vi "MasterAquisitionFile_IOS_US.vi"() -> ()   [LabVIEW 2018]
uses:
  <vilib>/userdefined/High Color/IMAQdx.ctl
  <vilib>/vision/driver/IMAQdx.llb/IMAQdx Camera Control Mode.ctl
  <vilib>/vision/driver/IMAQdx.llb/IMAQdx Acquisition Mode.ctl
  <vilib>/vision/driver/IMAQdx.llb/IMAQdx Buffer Number Mode.ctl
  <vilib>/DAQmx/write.llb/DAQmx Write (Digital Bool 1Line 1Point).vi
  <vilib>/DAQmx/read.llb/DAQmx Read (Analog 1D Wfm NChan NSamp).vi
  <vilib>/DAQmx/write.llb/DAQmx Write (Digital 1D Bool NChan 1Samp 1Line).vi
  <vilib>/DAQmx/create/channels.llb/DAQmx Create Channel (DO-Digital Output).vi
  <vilib>/DAQmx/create/channels.llb/DAQmx Create Channel (CO-Pulse Generation-Frequency).vi
  <vilib>/DAQmx/configure/timing.llb/DAQmx Timing (Implicit).vi
  <vilib>/DAQmx/create/channels.llb/DAQmx Create Channel (AI-Voltage-Basic).vi
  <vilib>/DAQmx/configure/timing.llb/DAQmx Timing (Sample Clock).vi
  <vilib>/DAQmx/configure/trigger.llb/DAQmx Start Trigger (Digital Edge).vi
  <vilib>/DAQmx/miscellaneous.llb/DAQmx Fill In Error Info.vi
  <vilib>/vision/driver/NI_Vision_Acquisition_Software.lvlib
  <resource>/objmgr/imaqdx.rc
panel:
  out "?":T1(plugin-control)
  out "?":T1(plugin-control)
  out "?":T1(plugin-control)
  in  "stop":bool
  out "CBV Cam":bool=TRUE
  out "Whisk Cam":bool=TRUE
  out "Web Cam":bool=TRUE
  out "Analog Data":bool=TRUE
  in  "Physical channels":tag="Dev1/ai0:7"
  out "Web Cam Fs":dbl(knob)=29.663547680668923 scale=0.0..200.0
  out "CBV Cam":dbl(knob)=30.019685039370078 scale=0.0..200.0
  out "Whisk Cam Fs":dbl(knob)=150.04985044865404 scale=0.0..200.0
  in  "Exposure Time (microsec)":string="10000"
  out "Solenoids":bool[](array[boolean])
  out "Analog Samples":i32=18000000
  in  "Analog Channels":string[](array[string])=["Cortical_LH", "Force_Sensor", "LPadSol", "RPadSol", "AudSol", "Hippocampus", "EMG", "Cortical_RH"]
  in  "Whisker Cam ID":T2="cam1"
  in  "WebCam ID":T2="cam0"
  in  "Analog Acquisition":cluster{"Analog Fs":u16}={"Analog Fs"=20000} {"Analog Fs" format="%0.0f"}
  in  "Camera Acquisition Setup":T3={"CBV Cam Fs"=30, "Whisk Cam Fs"=150, "Web Cam Fs"=15, "Pupil Cam Fs"=30}
  out "Notes Size":i32=7
  out "Notes Reversed":string[](array[string])=["Experimenter", "Animal ID", "Hemisphere", "Solenoid PSI", "Isoflurane time", "Session ID", "Amplifier Gain"]
  out "Notes Array":string[](array[string])=["Amplifier Gain", "Session ID", "Isoflurane time", "Solenoid PSI", "Hemisphere", "Animal ID", "Experimenter"]
  in  "Notes:":T4={"Experimenter"="Kevin", "Animal ID"="T119", "Hemisphere"="Both", "Solenoid PSI"="10", "Isoflurane time"="1000", "Session ID"="Imaging Session Six", "Amplifier Gain"="10000"}
  in  "Whisk Cam Trig Source":tag="Dev1/ctr1"
  in  "CBV Cam Trig Source":tag="Dev1/ctr0"
  in  "Right Pad":tag="Dev1/port0/line0"
  in  "Left Pad":tag="Dev1/port0/line1"
  in  "Ultrasound":tag="Dev1/port0/line2"
  in  "Offset (s)":dbl=15.0
  in  "Duration (s)":dbl=0.1 step=0.1
  in  "Interval (s)":dbl=30.0
  in  "Right Pad":dbl=1.0
  in  "Left Pad":dbl=1.0
  in  "Auditory":dbl=1.0
  in  "Target Path":path=path "D:/T119/Imaging Session 6 - 1.29.20" caption="Final saved file location"
  out "Dropped":u32(slide)=135 caption="Whisk Cam" scale=0.0..450.0
  out "Current file name":string="200128_14_10_25"
  out "CBV Camera":bool=TRUE
  out "Time Elapsed (Min)":cluster{dbl, dbl}(slide)={15.0, 15.00305001} scale=0.0..15.0 scale format="%#_2g"
  in  "Time (min)":dbl(knob)=15.0 min=0.5 max=20.0 step=0.5 scale=0.0..20.0 scale format="%#_2g"
  in  "Temp Path":path=path "D:/LabVIEW Streamed Data" caption="Temporary path for streamed data"
  out "Last CBV\nBuffer":i32=27000
  out "Last Whisk\nBuffer":u32=134865
  # "Stimuli"
  # "LPAD"
  # "RPAD"
  # "US"
  # "Whisk Cam ID"
  # "Ratio"
  # "Web Cam ID"
  # "Data Sampling Rates"
  # "Ratio"
  # "Ratio"
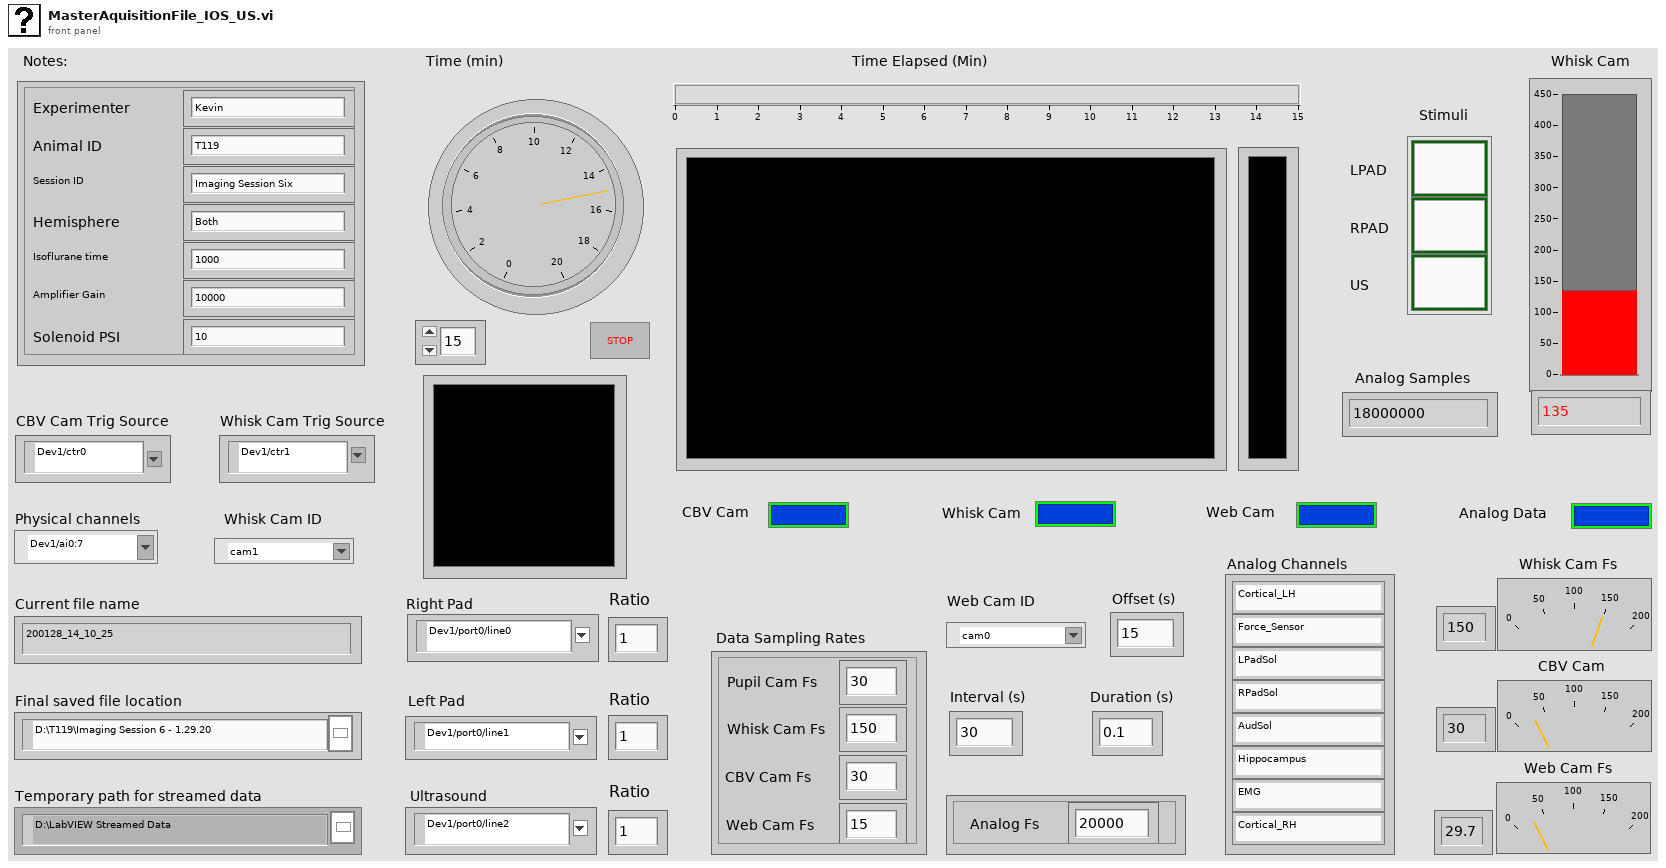
[diagram p1: front panel]
types:
  T1 = typedef "IMAQ Image.ctl" = refnum<image>
  T2 = typedef "IMAQdx.ctl" = refnum<k21>
  T3 = cluster{"CBV Cam Fs":u16, "Whisk Cam Fs":u16, "Web Cam Fs":u16, "Pupil Cam Fs":u16}
  T4 = cluster{"Experimenter":string, "Animal ID":string, "Hemisphere":string, "Solenoid PSI":string, "Isoflurane time":string, "Session ID":string, "Amplifier Gain":string}
  T5 = enum16{"open", "open or create", "create or replace", "create", "open (read-only)"}
  T6 = typedef "Image Type" = u32
  T7 = typedef "NI_Vision_Acquisition_Software.lvlib/IMAQdx Camera Control Mode.ctl" = enum32{"Controller", "Listener"}
  T8 = enum16{"open", "replace", "create", "open or create", "replace or create", "replace or create with confirmation"}
  T9 = typedef "NI_Vision_Acquisition_Software.lvlib/IMAQdx Acquisition Mode.ctl" = enum32{"One Shot", "Continuous"}
  T10 = typedef "IMAQ AVI2 Refnum.ctl" = refnum<k20>
  T11 = enum16{"big-endian, network order", "native, host order", "little-endian"}
  T12 = typedef "NI_Vision_Acquisition_Software.lvlib/IMAQdx Buffer Number Mode.ctl" = enum32{"Next", "Last", "Buffer Number", "Every", "Last New"}
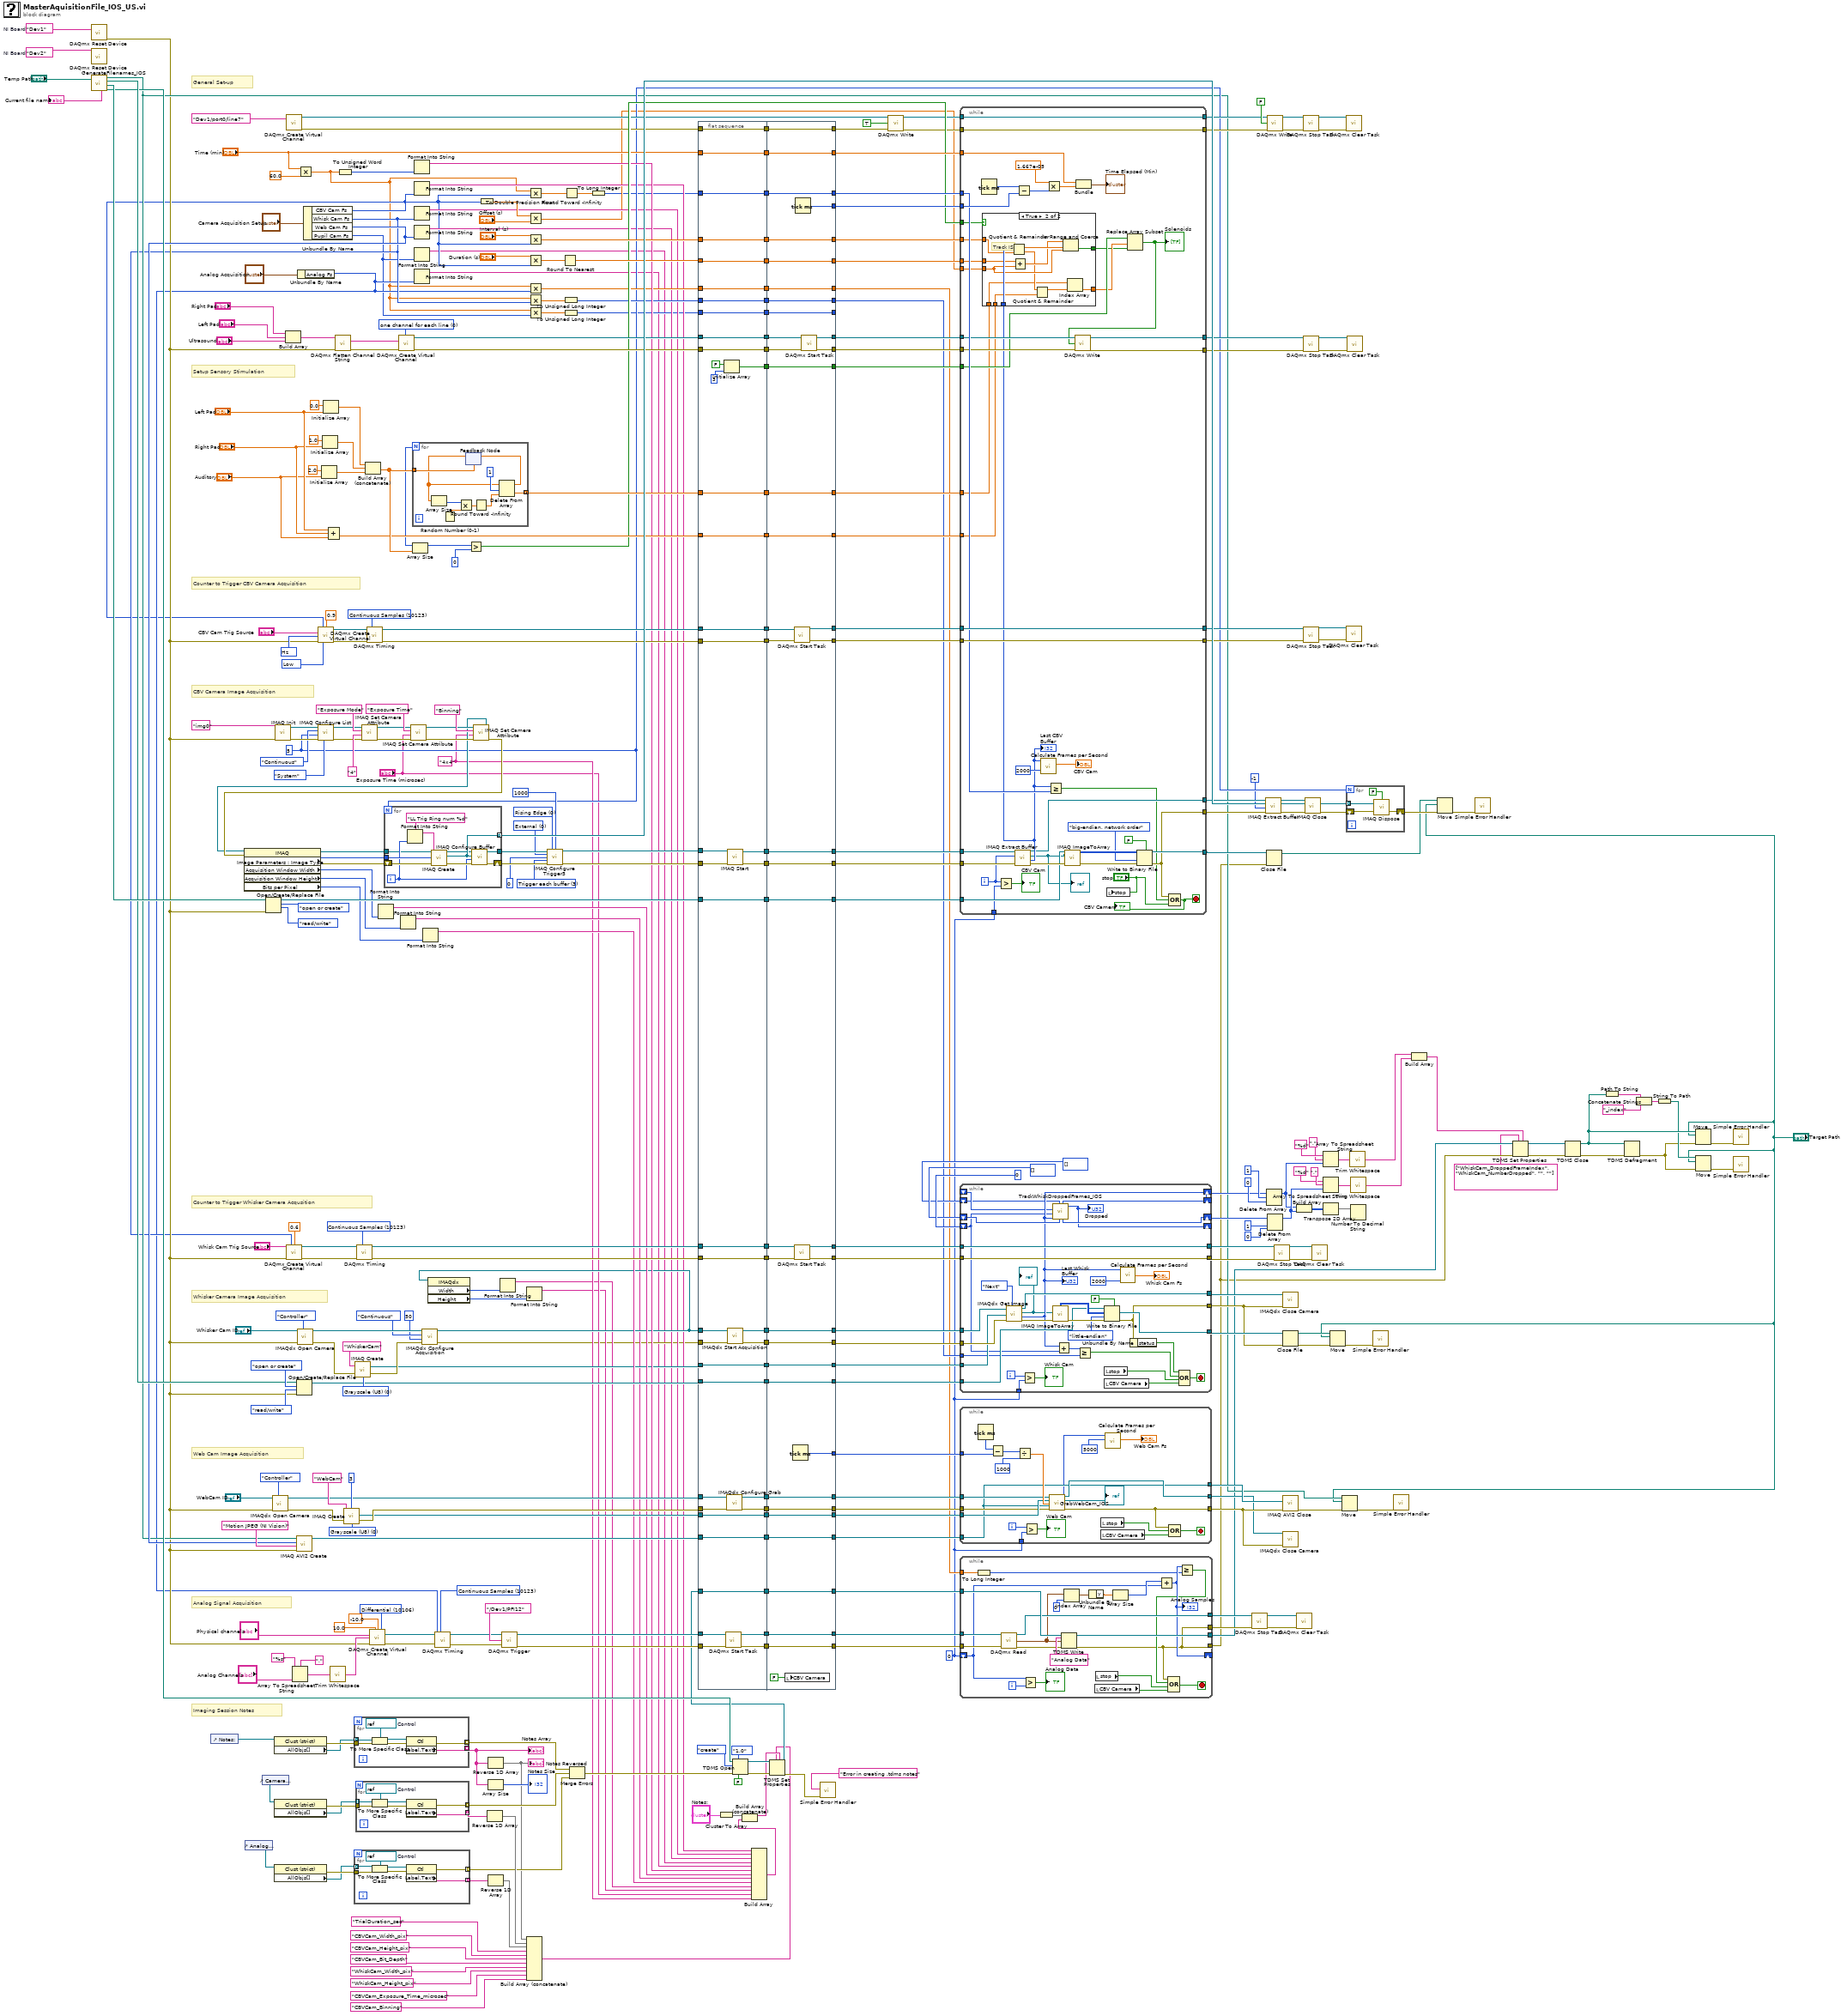
[diagram p0: block diagram]
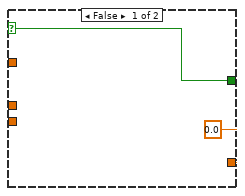
[diagram p2: hidden frame]
diagram:
  w16 = tag "Dev2"  # NI Board
  w48 = "4x4" ("Attribute Value")
  w22 = 0
  w207 = 0 items=["one channel for each line", "one channel for all lines"] ("line grouping")
  w260 = 10123 items=["Finite Samples"=10178, "Continuous Samples"=10123, "Hardware Timed Single Point"=12522] ("sample mode")
  w263 = 10106 items=["default"=-1, "RSE"=10083, "NRSE"=10078, "Differential"=10106, "Pseudodifferential"=12529] ("input terminal configuration")
  w314 = T6 0 items=["Grayscale (U8)", "Grayscale (I16)", "Grayscale (SGL)", "Complex (CSG)", "RGB (U32)", "HSL (U32)", "RGB (U64)", "Grayscale (U16)"] ("Image Type")
  w334 = u32 0 items=["Rising Edge", "Falling Edge"] ("Trigger Polarity")
  w337 = u32 0 items=["External"=0, "RTSI"=1, "ISO In"=2, "Scaled Encoder"=5] ("Trigger Type")
  w328 = tag "Dev1"  # NI Board
  w329 = 10123 items=["Finite Samples"=10178, "Continuous Samples"=10123, "Hardware Timed Single Point"=12522] ("sample mode")
  w332 = 10373 items=["Hz"=10373] ("units")
  w333 = 10214 items=["High"=10192, "Low"=10214] ("idle state")
  w53 = u32 5 ("Number of Buffers")
  w335 = u32 3 items=["Disabled", "Trigger start of acquisition", "Trigger start of each buffer list", "Trigger each buffer", "Trigger each line (linescan)", "Trigger end of acquisition"] ("Action")
  w349 = 10123 items=["Finite Samples"=10178, "Continuous Samples"=10123, "Hardware Timed Single Point"=12522] ("sample mode")
  w356 = T6 0 items=["Grayscale (U8)", "Grayscale (I16)", "Grayscale (SGL)", "Complex (CSG)", "RGB (U32)", "HSL (U32)", "RGB (U64)", "Grayscale (U16)"] ("Image Type")
  # "General Set-up"
  # "Whisker Camera Image Acquisition"
  # "Imaging Session Notes"
  # "Setup Sensory Stimulation"
  # "CBV Camera Image Acquisition"
  # "Counter to Trigger CBV Camera Acquisition"
  # "Counter to Trigger Whisker Camera Acqusition"
  # "Web Cam Image Acquisition"
  # "Analog Signal Acquisition"
  n1 = call <vilib>:"DAQmx Reset Device.vi"("device in"=w328) -> ("error out"=w44:errorcluster)  [unwired: 14 in]
  n2 = call <vilib>:"DAQmx Reset Device.vi"("device in"=w16) -> ()  [unwired: 14 in, 1 out]
  n3 = call "GenerateFilenames_IOS.vi"("path"="Temp Path") -> ("TDMS Path"=w163:path, "Dalsa Path"=w321:path, "Basler Path"=w317:path, "WebCam Path"=w52:path, "Analog file name"=→"Current file name":string)  [unwired: 3 in, 3 out]
  n4 = control-ref of="Notes:"() -> (w168:refnum<vi>)
  n5 = control-ref of="Analog Acquisition"() -> (w146:refnum<vi>)
  n6 = control-ref of="Camera Acquisition Setup"() -> (w147:refnum<vi>)
  n7 = Open/Create/Replace File(file path (use dialog)=w321, error in=w44, operation (0:open)=T8."open or create", access (0:read/write)=enum16{"read/write", "read-only", "write-only"}."read/write") -> (refnum out=w264:refnum<file>)  [unwired: 2 in, 2 out]
  n8 = call <vilib>:"IMAQdx Open Camera.vi"("Camera Control Mode"=IMAQdx_Camera_Control_Mode."Controller", "error in"=w44, "Session In"="WebCam ID") -> ("error out"=w310:errorcluster, "Session Out"=w308:T2)  [unwired: 7 in]
  n9 = property class="Clust (strict)"(reference=w168) -> (error out=w171:errorcluster, "AllObjs[]"=w60:refnum<vi>[])  [unwired: 1 in, 1 out]
  n10 = property class="Clust (strict)"(reference=w147) -> (error out=w166:errorcluster, "AllObjs[]"=w61:refnum<vi>[])  [unwired: 1 in, 1 out]
  n11 = property class="Clust (strict)"(reference=w146) -> (error out=w145:errorcluster, "AllObjs[]"=w59:refnum<vi>[])  [unwired: 1 in, 1 out]
  n12 = call <vilib>:"IMAQ Init.vi"("error in (no error)"=w44, "Interface Name"="img0") -> ("error out"=w347:errorcluster, "IMAQ Session Out"=w348:refnum<k11>)  [unwired: 8 out]
  n13 = Build Array("Right Pad", "Left Pad", "Ultrasound") -> (w11:tag[])
  n14 = call-poly <vilib>:"DAQmx Create Virtual Channel.vi"("lines"=tag "Dev1/port0/line7") -> ("task out"=w93:refnum<k21>, "error out"=w96:errorcluster)  [unwired: 13 in]
  n15 = Array To Spreadsheet String(delimiter (Tab)=",", array="Analog Channels", 3:"%s" ("format string")) -> (spreadsheet string=w132:string)
  n16 = Open/Create/Replace File(file path (use dialog)=w317, error in=w44, operation (0:open)=T8."open or create", access (0:read/write)=enum16{"read/write", "read-only", "write-only"}."read/write") -> (refnum out=w282:refnum<file>)  [unwired: 2 in, 2 out]
  n17 = Unbundle By Name("Analog Acquisition") -> ("Analog Fs"=w37:u16)
  n18 = call <vilib>:"IMAQdx Open Camera.vi"("Camera Control Mode"=IMAQdx_Camera_Control_Mode."Controller", "error in"=w44, "Session In"="Whisker Cam ID") -> ("error out"=w359:errorcluster, "Session Out"=w362:T2)  [unwired: 7 in]
  n19 = Multiply(x="Time (min)", y=60.0) -> (x*y=w24:dbl)
  n20 = Unbundle By Name("Camera Acquisition Setup") -> ("CBV Cam Fs"=w26:u16, "Whisk Cam Fs"=w42:u16, "Web Cam Fs"=w140:u16, "Pupil Cam Fs"=w35:u16)
  n21 = call-poly <vilib>:"DAQmx Create Virtual Channel.vi"("frequency"=w42, "duty cycle"=0.6, "counter"="Whisk Cam Trig Source", "error in"=w44) -> ("task out"=w351:refnum<k21>, "error out"=w350:errorcluster)  [unwired: 10 in]
  n22 = call "IMAQ AVI2 Create"("error in (no error)"=w44, "Codec"="Motion JPEG (NI Vision)", "Frames Per Second"=w140, "AVI Path"=w52) -> ("AVI Refnum"=w300:T10)  [unwired: 6 in, 1 out]
  n23 = call <vilib>:"IMAQ Configure List.vi"("Memory Location"=enum16{"System", "Onboard"}."System", "error in (no error)"=w347, "Number of buffers"=w53, "Continuous?"=enum16{"One-Shot", "Continuous"}."Continuous" ("Continuous ?"), "IMAQ Session In"=w348) -> ("error out"=w74:errorcluster, "IMAQ Session Out"=w70:refnum<k11>)  [unwired: 1 in, 4 out]
  n24 = call-poly <vilib>:"DAQmx Create Virtual Channel.vi"("frequency"=w26, "duty cycle"=0.9, "counter"="CBV Cam Trig Source", "units"=w332, "error in"=w44, "idle state"=w333) -> ("task out"=w331:refnum<k21>, "error out"=w330:errorcluster)  [unwired: 8 in]
  n25 = Initialize Array(2.0 ("element"), "Auditory") -> (w20:dbl[])
  n26 = Initialize Array(1.0 ("element"), "Right Pad") -> (w211:dbl[])
  n27 = Initialize Array(0.0 ("element"), "Left Pad") -> (w212:dbl[])
  n28 = Compound Arithmetic op=ADD("Left Pad", "Right Pad", "Auditory") -> (w191:dbl)
  n29 = call <vilib>:"Trim Whitespace.vi"("string"=w132) -> ("trimmed string"=w131:string)  [unwired: 1 in]
  n30 = call <vilib>:"DAQmx Flatten Channel String.vi"("names in"=w11, "error in"=w44) -> ("names out"=w173:string, "error out"=w172:errorcluster)  [unwired: 12 in]
  n31 = To Unsigned Word Integer(number=w24) -> (unsigned 16bit integer=w126:u16)
  n32 = call "IMAQ Create"("Border Size"=3, "Image Name"="WebCam", "Image Type"=w314, "error in (no error)"=w310) -> ("New Image"=w307:T1, "error out"=w309:errorcluster)  [unwired: 1 in]
  n33 = for {
    tunnel: [w368] -> w170 mode=indexing
    tunnel: w171 -> [w367]
    tunnel: [w365] -> w154 mode=indexing
    tunnel: w60 -> [w364] mode=indexing
    w369 = refnum<vi> refnum  # Control
    n34 = To More Specific Class(target class=w369, reference=w364, error in=w367) -> (specific class reference=w370:refnum<vi>, error out=w366:errorcluster)
    n35 = property class="Ctl"(reference=w370, error in=w366) -> (error out=w365:errorcluster, "Label.Text"=w368:string)  [unwired: 1 out]
  }
  "Notes Array" <- w170
  n36 = for {
    tunnel: [w375] -> w143 mode=indexing
    tunnel: w145 -> [w374]
    tunnel: [w372] -> w144 mode=indexing
    tunnel: w59 -> [w371] mode=indexing
    w376 = refnum<vi> refnum  # Control
    n37 = To More Specific Class(target class=w376, reference=w371, error in=w374) -> (specific class reference=w377:refnum<vi>, error out=w373:errorcluster)
    n38 = property class="Ctl"(reference=w377, error in=w373) -> (error out=w372:errorcluster, "Label.Text"=w375:string)  [unwired: 1 out]
  }
  n39 = call "IMAQ Create"("Image Name"="WhiskerCam", "Image Type"=w356, "error in (no error)"=w359) -> ("New Image"=w113:T1, "error out"=w357:errorcluster)  [unwired: 2 in]
  n40 = for {
    tunnel: [w382] -> w167 mode=indexing
    tunnel: w166 -> [w381]
    tunnel: [w379] -> w153 mode=indexing
    tunnel: w61 -> [w378] mode=indexing
    w383 = refnum<vi> refnum  # Control
    n41 = To More Specific Class(target class=w383, reference=w378, error in=w381) -> (specific class reference=w384:refnum<vi>, error out=w380:errorcluster)
    n42 = property class="Ctl"(reference=w384, error in=w380) -> (error out=w379:errorcluster, "Label.Text"=w382:string)  [unwired: 1 out]
  }
  n43 = call-poly <vilib>:"DAQmx Timing.vi"("task/channels in"=w351, "sample mode"=w349, "error in"=w350) -> ("task out"=w243:refnum<k21>, "error out"=w241:errorcluster)  [unwired: 11 in]
  n44 = call <vilib>:"IMAQ Set Camera Attribute.vi"("error in (no error)"=w74, "Attribute Value"="4", "Camera Attribute"="Exposure Mode", "IMAQ Session In"=w70) -> ("error out"=w73:errorcluster, "IMAQ Session Out"=w69:refnum<k11>)  [unwired: 4 in]
  n45 = Build Array (concatenate)(w212, w211, w20) -> (w210:dbl[])
  n46 = call-poly <vilib>:"DAQmx Timing.vi"("task/channels in"=w331, "sample mode"=w329, "error in"=w330) -> ("task out"=w247:refnum<k21>, "error out"=w245:errorcluster)  [unwired: 11 in]
  n47 = call-poly <vilib>:"DAQmx Create Virtual Channel.vi"("maximum value"=10.0, "minimum value"=-10.0, "input terminal configuration"=w263, "physical channels"="Physical channels", "name to assign"=w131, "error in"=w44) -> ("task out"=w262:refnum<k21>, "error out"=w261:errorcluster)  [unwired: 8 in]
  n48 = call-poly <vilib>:"DAQmx Create Virtual Channel.vi"("lines"=w173, "line grouping"=w207, "error in"=w172) -> ("task out"=w205:refnum<k21>, "error out"=w203:errorcluster)  [unwired: 11 in]
  n49 = call <vilib>:"IMAQ Set Camera Attribute.vi"("error in (no error)"=w73, "Attribute Value"="Exposure Time (microsec)", "Camera Attribute"="Exposure Time", "IMAQ Session In"=w69) -> ("error out"=w72:errorcluster, "IMAQ Session Out"=w68:refnum<k11>)  [unwired: 4 in]
  n50 = Array Size(array=w210) -> (size(s)=w137:i32)
  n51 = for {
    N: w137 -> [_]
    tunnel: w210 -> [w388]
    tunnel: [w385] -> w188 mode=concatenating
    n52 = Random Number (0-1)() -> (number: 0 to 1=w392:dbl)
    n53 = feedback #1(w388) -> (w387:dbl[])
    n54 = Array Size(array=w387) -> (size(s)=w393:i32)
    n55 = Multiply(x=w393, y=w392) -> (x*y=w391:dbl)
    n56 = Round Toward -Infinity(1:w391) -> (0:w390:dbl)
    n57 = Delete From Array(array=w387, length=1, index=w390) -> (deleted portion=w385:dbl[], array with subset deleted=w386:dbl[])
    n58 = feedback-in #1(w386) -> ()
  }
  n59 = Format Into String(w126) -> (resulting string=w128:string)  [unwired: 3 in, 1 out]
  n60 = Format Into String(w26) -> (resulting string=w40:string)  [unwired: 3 in, 1 out]
  n61 = Format Into String(w42) -> (resulting string=w39:string)  [unwired: 3 in, 1 out]
  n62 = Format Into String(w140) -> (resulting string=w38:string)  [unwired: 3 in, 1 out]
  n63 = Format Into String(w35) -> (resulting string=w6:string)  [unwired: 3 in, 1 out]
  n64 = Format Into String(w37) -> (resulting string=w5:string)  [unwired: 3 in, 1 out]
  n65 = call <vilib>:"IMAQdx Configure Acquisition.vi"("error in"=w357, "Number of Buffers"=u32 50, "Continuous?"=IMAQdx_Acquisition_Mode."Continuous", "Session In"=w362) -> ("error out"=w23:errorcluster, "Session Out"=w114:T2)  [unwired: 6 in]
  n66 = property class="IMAQdx"(reference=w114) -> ("Width"=w125:u32, "Height"=w124:u32)  [unwired: 1 in, 2 out]
  n67 = call-poly <vilib>:"DAQmx Timing.vi"("task/channels in"=w262, "sample mode"=w260, "rate"=w37, "error in"=w261) -> ("task out"=w57:refnum<k21>, "error out"=w259:errorcluster)  [unwired: 10 in]
  n68 = Greater?(x=w137, y=0) -> (0:w135:bool)
  n69 = call <vilib>:"IMAQ Set Camera Attribute.vi"("error in (no error)"=w72, "Attribute Value"=w48, "Camera Attribute"="Binning", "IMAQ Session In"=w68) -> ("error out"=w71:errorcluster, "IMAQ Session Out"=w67:refnum<k11>)  [unwired: 4 in]
  n70 = property class="IMAQ"(reference=w67, error in=w71) -> (reference out=w81:refnum<k11>, error out=w80:errorcluster, "Image Parameters : Image Type"=w343:u32, "Acquisition Window Width"=w123:u32, "Acquisition Window Height"=w122:u32, "Bits per Pixel"=w121:u32)
  n71 = Format Into String(w123) -> (resulting string=w120:string)  [unwired: 3 in, 1 out]
  n72 = for {
    N: w53 -> [_]
    tunnel: [w403] -> w339
    tunnel: w343 -> [w401]
    shift-right: [w402] -> w338
    shift-left: w80 -> [w400]
    tunnel: [w395] -> w340 mode=indexing
    tunnel: w81 -> [w394]
    i -> [w396]
    n73 = Format Into String(format string="LL Trig Ring num %d", w396) -> (resulting string=w398:string)  [unwired: 2 in, 1 out]
    n74 = call "IMAQ Create"("Image Name"=w398, "Image Type"=w401, "error in (no error)"=w400) -> ("New Image"=w395:T1, "error out"=w399:errorcluster)  [unwired: 1 in, 1 out]
    n75 = call <vilib>:"IMAQ Configure Buffer.vi"("error in (no error)"=w399, "Buffer Number"=w396, "Image In"=w395, "IMAQ Session In"=w394) -> ("error out"=w402:errorcluster, "IMAQ Session Out"=w403:refnum<k11>)  [unwired: 2 in, 4 out]
  }
  n76 = Format Into String(w122) -> (resulting string=w54:string)  [unwired: 3 in, 1 out]
  n77 = Format Into String(w121) -> (resulting string=w119:string)  [unwired: 3 in, 1 out]
  n78 = To Double Precision Float(number=w26) -> (double precision float=w174:dbl)
  n79 = Reverse 1D Array(array=w167) -> (reversed array=w157:string[])
  n80 = Reverse 1D Array(array=w170) -> (reversed array=w58:string[])
  "Notes Reversed" <- w58
  n81 = Array Size(array=w170) -> (size(s)=→"Notes Size":i32)
  n82 = Reverse 1D Array(array=w143) -> (reversed array=w142:string[])
  n83 = Format Into String(w125) -> (resulting string=w45:string)  [unwired: 3 in, 1 out]
  n84 = call-poly <vilib>:"DAQmx Trigger.vi"("task/channels in"=w57, "source"=tag "/Dev1/PFI12", "error in"=w259) -> ("task out"=w257:refnum<k21>, "error out"=w256:errorcluster)  [unwired: 11 in]
  n85 = Build Array (concatenate)(w58, w157, w142, "TrialDuration_sec", "CBVCam_Width_pix", "CBVCam_Height_pix", "CBVCam_Bit_Depth", "WhiskCam_Width_pix", "WhiskCam_Height_pix", "CBVCam_Exposure_Time_microsec" ("element"), "CBVCam_Binning" ("element")) -> (w49:string[])
  n86 = Format Into String(w124) -> (resulting string=w46:string)  [unwired: 3 in, 1 out]
  n87 = Multiply(x=w24, y=w26) -> (x*y=w319:dbl)
  n88 = Multiply(x="Offset (s)", y=w174) -> (x*y=w33:dbl)
  n89 = Multiply(x="Interval (s)", y=w26) -> (x*y=w195:dbl)
  n90 = Multiply(x="Duration (s)", y=w26) -> (x*y=w182:dbl)
  n91 = Multiply(x=w24, y=w37) -> (x*y=w102:dbl)
  n92 = Multiply(x=w42, y=w24) -> (x*y=w55:dbl)
  n93 = Multiply(x=w35, y=w24) -> (x*y=w41:dbl)
  n94 = call <vilib>:"IMAQ Configure Trigger3.vi"("IMAQ Session In"=w339, "Polarity"=w334, "Frame timeout (ms)"=u32 1000 ("Frame Timeout (ms)"), "Type"=w337, "Line Number"=u32 0 ("Trigger Line Number"), "Action"=w335, "error in (no error)"=w338) -> ("IMAQ Session Out"=w281:refnum<k11>, "error out"=w280:errorcluster)  [unwired: 2 in, 5 out]
  n95 = Round To Nearest(number=w182) -> (nearest integer value=w181:dbl)
  n96 = To Unsigned Long Integer(number=w55) -> (unsigned 32bit integer=w100:u32)
  n97 = To Unsigned Long Integer(number=w41) -> (unsigned 32bit integer=w36:u32)
  n98 = Round Toward -Infinity(1:w319) -> (0:w318:dbl)
  n99 = Merge Errors(w154, w153, w144) -> (w152:errorcluster)
  n100 = To Long Integer(number=w318) -> (32bit integer=w25:i32)
  n101 = flat-sequence {
    tunnel: w309 -> [w444]
    tunnel: w308 -> [w443]
    tunnel: w307 -> [w442]
    tunnel: [w442] -> w306
    tunnel: [w441] -> w304
    tunnel: [w440] -> w302
    tunnel: w300 -> [w439]
    tunnel: [w439] -> w299
    tunnel: w114 -> [w438]
    tunnel: w23 -> [w437]
    tunnel: [w436] -> w289
    tunnel: [w435] -> w287
    tunnel: [w434] -> w285
    tunnel: w113 -> [w434]
    tunnel: [w433] -> w283
    tunnel: w282 -> [w433]
    tunnel: w281 -> [w432]
    tunnel: w280 -> [w431]
    tunnel: [w430] -> w278
    tunnel: [w429] -> w276
    tunnel: w25 -> [w428]
    tunnel: [w428] -> w270
    tunnel: "Time (min)" -> [w427]
    tunnel: [w427] -> w267
    tunnel: [w426] -> w265
    tunnel: w264 -> [w426]
    tunnel: w257 -> [w425]
    tunnel: w256 -> [w424]
    tunnel: [w423] -> w255
    tunnel: [w422] -> w254
    tunnel: [w421] -> w249
    tunnel: w155 -> [w421]
    tunnel: w247 -> [w420]
    tunnel: [w420] -> w246
    tunnel: w245 -> [w419]
    tunnel: [w419] -> w244
    tunnel: w243 -> [w418]
    tunnel: [w418] -> w242
    tunnel: w241 -> [w417]
    tunnel: [w417] -> w240
    tunnel: w205 -> [w416]
    tunnel: [w416] -> w206
    tunnel: w203 -> [w415]
    tunnel: [w415] -> w204
    tunnel: w195 -> [w414]
    tunnel: [w414] -> w194
    tunnel: [w413] -> w192
    tunnel: w181 -> [w413]
    tunnel: w191 -> [w412]
    tunnel: [w412] -> w190
    tunnel: w188 -> [w411]
    tunnel: [w411] -> w187
    tunnel: [w409] -> w185
    tunnel: w102 -> [w407]
    tunnel: [w407] -> w101
    tunnel: w100 -> [w406]
    tunnel: [w406] -> w99
    tunnel: w96 -> [w405]
    tunnel: [w405] -> w95
    tunnel: w36 -> [w404]
    tunnel: [w404] -> w34
    tunnel: [w484] -> w311
    tunnel: w306 -> [w483]
    tunnel: [w483] -> w305
    tunnel: w304 -> [w482]
    tunnel: [w482] -> w303
    tunnel: w302 -> [w481]
    tunnel: [w481] -> w301
    tunnel: w299 -> [w480]
    tunnel: [w480] -> w298
    tunnel: [w462] -> w295
    tunnel: [w461] -> w293
    tunnel: [w479] -> w290
    tunnel: w289 -> [w479]
    tunnel: [w478] -> w288
    tunnel: w287 -> [w478]
    tunnel: [w477] -> w286
    tunnel: w285 -> [w477]
    tunnel: [w476] -> w284
    tunnel: w283 -> [w476]
    tunnel: [w475] -> w279
    tunnel: w278 -> [w475]
    tunnel: [w474] -> w277
    tunnel: w276 -> [w474]
    tunnel: [w466] -> w274
    tunnel: [w465] -> w272
    tunnel: [w473] -> w271
    tunnel: w270 -> [w472]
    tunnel: [w472] -> w269
    tunnel: [w471] -> w268
    tunnel: w267 -> [w471]
    tunnel: [w470] -> w266
    tunnel: w265 -> [w470]
    tunnel: [w469] -> w252
    tunnel: w255 -> [w469]
    tunnel: [w468] -> w253
    tunnel: w254 -> [w468]
    tunnel: [w467] -> w250
    tunnel: w249 -> [w467]
    tunnel: w246 -> [w464]
    tunnel: w244 -> [w463]
    tunnel: w242 -> [w460]
    tunnel: w240 -> [w459]
    tunnel: w206 -> [w458]
    tunnel: w204 -> [w457]
    tunnel: [w456] -> w202
    tunnel: [w455] -> w201
    tunnel: [w454] -> w196
    tunnel: w194 -> [w454]
    tunnel: [w453] -> w193
    tunnel: w192 -> [w453]
    tunnel: w190 -> [w452]
    tunnel: [w452] -> w189
    tunnel: w187 -> [w451]
    tunnel: [w451] -> w186
    tunnel: w185 -> [w450]
    tunnel: [w450] -> w184
    tunnel: w101 -> [w449]
    tunnel: [w449] -> w31
    tunnel: w99 -> [w448]
    tunnel: [w448] -> w32
    tunnel: w95 -> [w447]
    tunnel: [w447] -> w94
    tunnel: [w445] -> _
    tunnel: w34 -> [w445]
    frame #0 {
      n102 = Initialize Array(FALSE, 3 ("dimension size")) -> (w409:bool[])
      n103 = call <vilib>:"DAQmx Start Task.vi"("task/channels in"=w425, "error in"=w424) -> ("task out"=w423:refnum<k21>, "error out"=w422:errorcluster)  [unwired: 12 in]
      n104 = call <vilib>:"IMAQdx Configure Grab.vi"("error in"=w444, "Session In"=w443) -> ("error out"=w440:errorcluster, "Session Out"=w441:T2)  [unwired: 8 in]
      n105 = call <vilib>:"IMAQ Start.vi"("error in (no error)"=w431, "IMAQ Session In"=w432) -> ("error out"=w429:errorcluster, "IMAQ Session Out"=w430:refnum<k11>)  [unwired: 8 out]
      n106 = call <vilib>:"IMAQdx Start Acquisition.vi"("error in"=w437, "Session In"=w438) -> ("error out"=w435:errorcluster, "Session Out"=w436:T2)  [unwired: 8 in]
    }
    frame #1 {
      n107 = local write "CBV Camera"(FALSE ("Finished Acquiring")) -> ()
      n108 = Tick Count (ms)() -> (millisecond timer value=w484:u32)
      n109 = call <vilib>:"DAQmx Start Task.vi"("task/channels in"=w464, "error in"=w463) -> ("task out"=w466:refnum<k21>, "error out"=w465:errorcluster)  [unwired: 12 in]
      n110 = call <vilib>:"DAQmx Start Task.vi"("task/channels in"=w460, "error in"=w459) -> ("task out"=w462:refnum<k21>, "error out"=w461:errorcluster)  [unwired: 12 in]
      n111 = Tick Count (ms)() -> (millisecond timer value=w473:u32)
      n112 = call <vilib>:"DAQmx Start Task.vi"("task/channels in"=w458, "error in"=w457) -> ("task out"=w456:refnum<k21>, "error out"=w455:errorcluster)  [unwired: 12 in]
    }
  }
  n113 = Cluster To Array(cluster="Notes:") -> (array=w164:string[])
  n114 = TDMS Open(6:FALSE ("disable buffering? (T)"), 7:enum16{"1.0", "2.0"}."1.0" ("file format version (2.0)"), 8:w152, 10:T5."create" ("operation (0:open)"), 11:w163) -> (0:w158:errorcluster, 3:w159:refnum<k34>)  [unwired: 2 in]
  n115 = Build Array(w40, w39, w38, w6, w5, w128, w120, w54, w119, w45, w46, "Exposure Time (microsec)", w48) -> (w139:string[])
  n116 = Build Array (concatenate)(w164, w139) -> (w156:string[])
  n117 = TDMS Set Properties(5:w156, 7:w49, 8:w158, 11:w159) -> (0:w151:errorcluster, 3:w155:refnum<k34>)  [unwired: 2 in, 2 out]
  n118 = call <vilib>:"Simple Error Handler.vi"("error source (\" \")"="Error in creating .tdms notes" ("error source (\" \")"), "error in (no error)"=w151) -> ()  [unwired: 3 in, 5 out]
  n119 = call-poly <vilib>:"DAQmx Write.vi"("task/channels in"=w93, "data"=TRUE, "error in"=w94) -> ("task out"=w91:refnum<k21>, "error out"=w89:errorcluster)  [unwired: 10 in, 1 out]
  n120 = while {
    tunnel: w279 -> [w530]
    tunnel: w277 -> [w531]
    tunnel: [w495] -> w323
    tunnel: [w493] -> w324
    tunnel: [w525] -> w322
    tunnel: [w520] -> w275
    tunnel: w274 -> [w520]
    tunnel: [w519] -> w273
    tunnel: w272 -> [w519]
    tunnel: w271 -> [w518]
    tunnel: w269 -> [w517]
    tunnel: w268 -> [w516]
    tunnel: w266 -> [w492]
    tunnel: w202 -> [w513]
    tunnel: w201 -> [w512]
    tunnel: [w511] -> w200
    tunnel: [w510] -> w199
    tunnel: w196 -> [w505]
    tunnel: w193 -> [w504]
    tunnel: w189 -> [w502]
    tunnel: w186 -> [w500]
    tunnel: w184 -> [w509]
    tunnel: w33 -> [w503]
    tunnel: w135 -> [w507]
    tunnel: w91 -> [w497]
    tunnel: [w497] -> w90
    tunnel: [w496] -> w88
    tunnel: w89 -> [w496]
    tunnel: w22 -> [w487]
    i -> [w488]
    stop <- w498 stop-if-true
    # "Track ISI"
    n121 = Tick Count (ms)() -> (millisecond timer value=w523:u32)
    n122 = Greater?(x=w488, y=w487) -> (0:→"CBV Cam":bool)
    n123 = call <vilib>:"IMAQ Extract Buffer.vi"("error in (no error)"=w531, "Buffer to extract"=w488, "IMAQ Session In"=w530) -> ("error out"=w524:errorcluster, "Buffer Number"=w506:i32, "Image Out"=w485:T1, "IMAQ Session Out"=w493:refnum<k11>)  [unwired: 5 out]
    "Last CBV\nBuffer" <- w506
    "?" <- w485
    n124 = case shown="True" w507 {
      selector: w507 -> [w533 _]
      tunnel: w506 -> [_ w543]
      tunnel: w505 -> [_ w542]
      tunnel: w504 -> [_ w541]
      tunnel: w503 -> [_ w540]
      tunnel: w502 -> [_ w537]
      tunnel: [0.0 ("element") w534] -> w501
      tunnel: w500 -> [_ w536]
      tunnel: [w533 w535] -> w499
      frame False {
      }
      frame True {
        n125 = Quotient & Remainder(x=w543, y=w542) -> (x-y*floor(x/y)=w545:dbl, floor(x/y)=w538:dbl)
        n126 = Add(x=w541, y=w540) -> (x+y=w544:dbl)
        n127 = Quotient & Remainder(x=w538, y=w537) -> (x-y*floor(x/y)=w539:dbl)  [unwired: 1 out]
        n128 = In Range and Coerce(upper limit=w544, x=w545, lower limit=w540) -> (In Range?=w535:bool)  [unwired: 1 out]
        n129 = Index Array(array=w536, index=w539) -> (element=w534:dbl)
      }
    }
    n130 = Subtract(x=w523, y=w518) -> (x-y=w522:u32)
    n131 = call <vilib>:"Calculate Frames per Second.vi"("Update Interval (ms)"=u32 2000, "Buffer Number"=w506) -> ("Processed Frames/s"=→"CBV Cam":dbl)  [unwired: 7 in, 2 out]
    n132 = Multiply(x=w522, y=1.667e-05) -> (x*y=w521:dbl)
    n133 = Greater Or Equal?(x=w506, y=w517) -> (x >= y?=w491:bool)
    n134 = call "IMAQ ImageToArray"("error in (no error)"=w524, "Image"=w485) -> ("error out"=w529:errorcluster, "Image Pixels (I16)"=w528:i16[][])  [unwired: 2 in, 3 out]
    n135 = Bundle("Time (min)"=w516, w521) -> (→"Time Elapsed (Min)":cluster{"Time (min)":dbl, dbl})  [unwired: 1 in]
    n136 = local write "stop"("stop") -> ()
    n137 = Replace Array Subset(array=w509, new element=w499, index=w501) -> (w508:bool[])
    "Solenoids" <- w508
    n138 = call-poly <vilib>:"DAQmx Write.vi"("task/channels in"=w513, "data"=w508, "error in"=w512) -> ("task out"=w511:refnum<k21>, "error out"=w510:errorcluster)  [unwired: 10 in, 1 out]
    n139 = Write to Binary File(file (use dialog)=w492, data=w528, error in=w529, 5:FALSE ("prepend array or string size? (T)"), 9:T11."big-endian, network order" ("byte order (0:big-endian, network order)")) -> (refnum out=w525:refnum<file>, error out=w495:errorcluster)  [unwired: 1 in, 1 out]
    n140 = Compound Arithmetic op=OR(w495, w491, "stop") -> (w498:bool)
    "CBV Camera" <- w498
  }
  n141 = while {
    tunnel: w295 -> [w573]
    tunnel: [w574] -> w294
    tunnel: w293 -> [w574]
    tunnel: [w573] -> w292
    tunnel: [w566] -> w111
    tunnel: [w567] -> w175
    tunnel: [w572] -> w291
    tunnel: w290 -> [w571]
    tunnel: w288 -> [w570]
    tunnel: w286 -> [w569]
    tunnel: w284 -> [w568]
    shift-right: [w554] -> _
    shift-left: _ -> [w552]
    shift-right: [w549] -> _
    shift-left: u32 0 ("New Lost") -> [w553]
    shift-right: [w550] -> w103
    shift-left: u32[] [] ("NewBuffNum") -> [w551]
    shift-right: [w556] -> w234
    shift-left: u32[] [] ("NewNumLost") -> [w555]
    tunnel: w32 -> [w564]
    tunnel: w22 -> [w557]
    i -> [w558]
    stop <- w561 stop-if-true
    n142 = call <vilib>:"IMAQdx Get Image.vi"("Buffer Number Mode (Next)"=IMAQdx_Buffer_Number_Mode."Next", "error in"=w570, "Image In"=w569, "Session In"=w571) -> ("error out"=w580:errorcluster, "Buffer Number Out"=w554:u32, "Image Out"=w546:T1, "Session Out"=w566:T2)  [unwired: 4 in]
    "Last Whisk\nBuffer" <- w554
    "?" <- w546
    n143 = Greater?(x=w558, y=w557) -> (0:→"Whisk Cam":bool)
    n144 = call "IMAQ ImageToArray"("error in (no error)"=w580, "Image"=w546) -> ("error out"=w579:errorcluster, "Image Pixels (U8)"=w578:u8[][])  [unwired: 2 in, 3 out]
    n145 = call "TrackWhiskDroppedFrames_IOS.vi"("NumLost"=w555, "BuffNum"=w551, "Curr Buffer"=w554, "Prev Lost"=w553, "Prev Buffer"=w552) -> ("New Lost"=w549:u32, "NewNumLost"=w556:u32[], "NewBuffNum"=w550:u32[])  [unwired: 4 in]
    "Dropped" <- w549
    n146 = Add(x=w554, y=w553) -> (x+y=w565:u32)
    n147 = Greater Or Equal?(x=w565, y=w564) -> (x >= y?=w562:bool)
    n148 = Write to Binary File(file (use dialog)=w568, data=w578, error in=w579, 5:FALSE ("prepend array or string size? (T)"), 9:T11."little-endian" ("byte order (0:big-endian, network order)")) -> (refnum out=w572:refnum<file>, error out=w567:errorcluster)  [unwired: 1 in, 1 out]
    n149 = local read "stop"() -> (w548:bool)
    n150 = local read "CBV Camera"() -> (w547:bool)
    n151 = call <vilib>:"Calculate Frames per Second.vi"("Update Interval (ms)"=u32 2000, "Buffer Number"=w554) -> ("Processed Frames/s"=→"Whisk Cam Fs":dbl)  [unwired: 7 in, 2 out]
    n152 = Unbundle By Name(w567) -> ("status"=w563:bool)
    n153 = Compound Arithmetic op=OR(w563, w562, w548, w547) -> (w561:bool)
  }
  n154 = while {
    tunnel: w311 -> [w598]
    tunnel: w305 -> [w596]
    tunnel: w303 -> [w595]
    tunnel: w301 -> [w594]
    tunnel: w298 -> [w592]
    tunnel: [w593] -> w43
    tunnel: [w584] -> w296
    tunnel: [w592] -> w297
    tunnel: w22 -> [w587]
    i -> [w588]
    stop <- w585 stop-if-true
    n155 = Tick Count (ms)() -> (millisecond timer value=w600:u32)
    n156 = Subtract(x=w600, y=w598) -> (x-y=w601:u32)
    n157 = Divide(x=w601, y=u32 1000) -> (x/y=w597:dbl)
    n158 = Greater?(x=w588, y=w587) -> (0:→"Web Cam":bool)
    n159 = call "GrabWebCam_IOS.vi"("Session In"=w595, "Image In"=w596, "Trial Time"=w597, "AVI Refnum"=w592, "error in"=w594) -> ("Session Out"=w593:T2, "WebCam Img Out"=→"?":T1, "Buffer Number Out"=w591:u32, "error out"=w584:errorcluster)  [unwired: 7 in]
    n160 = local read "CBV Camera"() -> (w586:bool)
    n161 = local read "stop"() -> (w583:bool)
    n162 = call <vilib>:"Calculate Frames per Second.vi"("Update Interval (ms)"=u32 5000, "Buffer Number"=w591) -> ("Processed Frames/s"=→"Web Cam Fs":dbl)  [unwired: 7 in, 2 out]
    n163 = Compound Arithmetic op=OR(w584, w583, w586) -> (w585:bool)
  }
  n164 = while {
    tunnel: w253 -> [w625]
    tunnel: w252 -> [w624]
    tunnel: w250 -> [w623]
    tunnel: [w622] -> w28
    tunnel: [w610] -> w27
    tunnel: [w621] -> w248
    shift-right: [w614] -> _
    shift-left: w22 -> [w605]
    tunnel: [w610] -> w50
    tunnel: w31 -> [w608]
    i -> [w606]
    stop <- w611 stop-if-true
    n165 = To Long Integer(number=w608) -> (32bit integer=w609:i32)
    n166 = call-poly <vilib>:"DAQmx Read.vi"("task/channels in"=w624, "error in"=w625) -> ("task out"=w621:refnum<k21>, "data"=w619:waveform(dbl)[], "error out"=w613:errorcluster)  [unwired: 11 in]
    n167 = Greater?(x=w605, y=w606) -> (0:→"Analog Data":bool)
    n168 = TDMS Write(0:w623, 5:"Analog Data" ("group name in (Untitled)"), 9:w619, 11:w613) -> (4:w622:refnum<k34>, 15:w610:errorcluster)  [unwired: 2 in, 2 out]
    n169 = Index Array(array=w619, index=0) -> (element=w617:waveform(dbl))
    n170 = Unbundle By Name(w617) -> ("Y"=w616:dbl[])
    n171 = local read "CBV Camera"() -> (w604:bool)
    n172 = local read "stop"() -> (w603:bool)
    n173 = Array Size(array=w616) -> (size(s)=w615:i32)
    n174 = Add(x=w615, y=w605) -> (x+y=w614:i32)
    "Analog Samples" <- w614
    n175 = Greater Or Equal?(x=w614, y=w609) -> (x >= y?=w612:bool)
    n176 = Compound Arithmetic op=OR(w610, w612, w603, w604) -> (w611:bool)
  }
  n177 = call <vilib>:"DAQmx Stop Task.vi"("task/channels in"=w248, "error in"=w50) -> ("task out"=w177:refnum<k21>, "error out"=w176:errorcluster)  [unwired: 12 in]
  n178 = call <vilib>:"IMAQ Extract Buffer.vi"("error in (no error)"=w323, "Buffer to extract"=-1, "IMAQ Session In"=w324) -> ("error out"=w345:errorcluster, "IMAQ Session Out"=w344:refnum<k11>)  [unwired: 7 out]
  n179 = Close File(refnum=w322, error in=w27) -> (path=w228:path)  [unwired: 1 out]
  n180 = Delete From Array(array=w103, length=1, index=0) -> (array with subset deleted=w63:u32[])  [unwired: 1 out]
  n181 = call-poly <vilib>:"DAQmx Write.vi"("task/channels in"=w90, "data"=FALSE, "error in"=w88) -> ("task out"=w87:refnum<k21>, "error out"=w85:errorcluster)  [unwired: 10 in, 1 out]
  n182 = Delete From Array(array=w234, length=1, index=0) -> (array with subset deleted=w64:u32[])  [unwired: 1 out]
  n183 = call <vilib>:"DAQmx Stop Task.vi"("task/channels in"=w292, "error in"=w294) -> ("task out"=w12:refnum<k21>, "error out"=w13:errorcluster)  [unwired: 12 in]
  n184 = call <vilib>:"IMAQdx Close Camera.vi"("error in"=w175, "Session In"=w111) -> ()  [unwired: 9 in, 1 out]
  n185 = Close File(refnum=w291, error in=w175) -> (path=w226:path, error out=w225:errorcluster)
  n186 = call "IMAQ AVI2 Close"("error in (no error)"=w296, "AVI Refnum"=w297) -> ("error out"=w227:errorcluster)  [unwired: 9 in]
  n187 = call <vilib>:"IMAQdx Close Camera.vi"("error in"=w296, "Session In"=w43) -> ()  [unwired: 9 in, 1 out]
  n188 = Build Array(w63, w64) -> (w66:u32[][])
  n189 = call <vilib>:"DAQmx Clear Task.vi"("task in"=w177, "error in"=w176) -> ()  [unwired: 13 in, 1 out]
  n190 = call <vilib>:"DAQmx Stop Task.vi"("task/channels in"=w87, "error in"=w85) -> ("task out"=w86:refnum<k21>, "error out"=w84:errorcluster)  [unwired: 12 in]
  n191 = call <vilib>:"DAQmx Stop Task.vi"("task/channels in"=w200, "error in"=w199) -> ("task out"=w198:refnum<k21>, "error out"=w197:errorcluster)  [unwired: 12 in]
  n192 = call <vilib>:"DAQmx Stop Task.vi"("task/channels in"=w275, "error in"=w273) -> ("task out"=w14:refnum<k21>, "error out"=w15:errorcluster)  [unwired: 12 in]
  n193 = call <vilib>:"IMAQ Close.vi"("error in (no error)"=w345, "IMAQ Session In"=w344) -> ("error out"=w346:errorcluster)  [unwired: 9 out]
  n194 = call <vilib>:"DAQmx Clear Task.vi"("task in"=w12, "error in"=w13) -> ()  [unwired: 13 in, 1 out]
  n195 = Array To Spreadsheet String(delimiter (Tab)=",", array=w64, 3:"%d" ("format string")) -> (spreadsheet string=w104:string)
  n196 = Transpose 2D Array(2D array=w66) -> (transposed array=w65:u32[][])
  n197 = Array To Spreadsheet String(delimiter (Tab)=",", array=w63, 3:"%d" ("format string")) -> (spreadsheet string=w105:string)
  n198 = Move(source path=w226, error in=w225, 10:"Target Path") -> (error out=w223:errorcluster)  [unwired: 2 in, 2 out]
  n199 = Move(source path=w52, error in=w227, 10:"Target Path") -> (error out=w222:errorcluster)  [unwired: 2 in, 2 out]
  n200 = call <vilib>:"DAQmx Clear Task.vi"("task in"=w14, "error in"=w15) -> ()  [unwired: 13 in, 1 out]
  n201 = call <vilib>:"DAQmx Clear Task.vi"("task in"=w86, "error in"=w84) -> ()  [unwired: 13 in, 1 out]
  n202 = for {
    N: w53 -> [_]
    tunnel: w340 -> [w629] mode=indexing
    shift-right: [w627] -> w230
    shift-left: w346 -> [w628]
    n203 = call "IMAQ Dispose"("All Images? (No)"=FALSE, "Image"=w629, "error in (no error)"=w628) -> ("error out"=w627:errorcluster)  [unwired: 3 out]
  }
  n204 = call <vilib>:"DAQmx Clear Task.vi"("task in"=w198, "error in"=w197) -> ()  [unwired: 13 in, 1 out]
  n205 = call <vilib>:"Trim Whitespace.vi"("string"=w105) -> ("trimmed string"=w9:string)  [unwired: 1 in]
  n206 = call <vilib>:"Trim Whitespace.vi"("string"=w104) -> ("trimmed string"=w8:string)  [unwired: 1 in]
  n207 = Number To Decimal String(number=w65) -> ()  [unwired: 1 in, 1 out]
  n208 = call <vilib>:"Simple Error Handler.vi"("error in (no error)"=w223) -> ()  [unwired: 1 in, 8 out]
  n209 = call <vilib>:"Simple Error Handler.vi"("error in (no error)"=w222) -> ()  [unwired: 1 in, 8 out]
  n210 = Build Array(w9, w8) -> (w7:string[])
  n211 = Move(source path=w228, error in=w230, 10:"Target Path") -> (error out=w229:errorcluster)  [unwired: 2 in, 2 out]
  n212 = call <vilib>:"Simple Error Handler.vi"("error in (no error)"=w229) -> ()  [unwired: 1 in, 8 out]
  n213 = TDMS Set Properties(5:w7, 7:string[] ["WhiskCam_DroppedFrameIndex", "WhiskCam_NumberDropped", "", ""] ("channel name(s) in (Untitled)"), 8:w27, 11:w28) -> (0:w112:errorcluster, 3:w110:refnum<k34>)  [unwired: 2 in, 2 out]
  n214 = TDMS Close(8:w112, 11:w110) -> (0:w231:errorcluster, 3:w219:path)
  n215 = Path To String(path=w219) -> (string=w221:string)
  n216 = TDMS Defragment(4:w231, 7:w219) -> (0:w216:errorcluster)
  n217 = Concatenate Strings(w221, "_index" ("string")) -> (w218:string)
  n218 = String To Path(string=w218) -> (path=w217:path)
  n219 = Move(source path=w219, error in=w216, 10:"Target Path") -> (error out=w224:errorcluster)  [unwired: 2 in, 2 out]
  n220 = Move(source path=w217, error in=w216, 10:"Target Path") -> (error out=w30:errorcluster)  [unwired: 2 in, 2 out]
  n221 = call <vilib>:"Simple Error Handler.vi"("error in (no error)"=w224) -> ()  [unwired: 1 in, 8 out]
  n222 = call <vilib>:"Simple Error Handler.vi"("error in (no error)"=w30) -> ()  [unwired: 1 in, 8 out]
